vi "Apply UI Theme.vi"(4 "close ref?":bool=TRUE, 6 "save?":bool=TRUE, 7 "VI Refnum":refnum<vi>, 8 "error in":errorcluster, 10 "Theme Mode":u16(ring)=3 items=["Light Theme", "Light Medium Contrast", "Light High Contrast", "Dark Theme", "Dark Medium Contrast", "Dark High Constrast"], 11 "Material Theme in":refnum<class "Material Theme.lvclass">) -> (0 "error out":errorcluster, 3 "Material Theme out":refnum<class "Material Theme.lvclass">)   [LabVIEW 2021, in "TSC Material Theme.lvlib" / "Material Theme.lvclass"]
doc: "Apply a loaded theme to a VI - will update the panel and the controls/indicators\n\n<b>Code Developed By:</b>\nDaniel Coons\nTechnology Service Corporation\nwww.tsc.com/atcs"
uses:
  Material Theme.lvclass
  <vilib>/Utility/traverseref.llb/TRef TravTarget.ctl
  Material Theme.lvclass/Material Theme.ctl
  Material-Scheme/Material-Scheme.lvclass
  <vilib>/Utility/traverseref.llb/VI Scripting - Traverse.lvlib
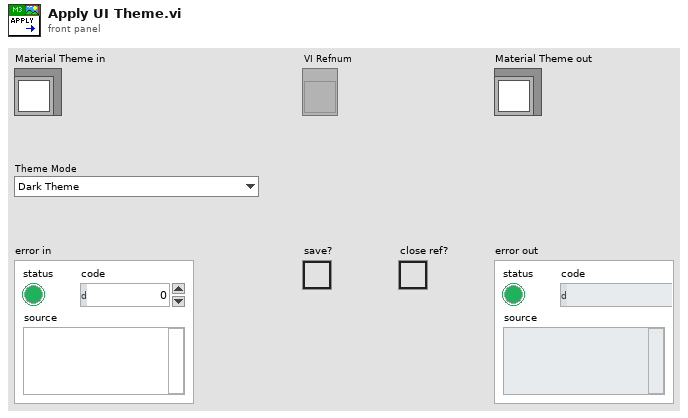
[diagram p1: front panel]
types:
  T1 = typedef "TRef TravTarget.ctl" = enum16{"FP", "BD", "Other"}
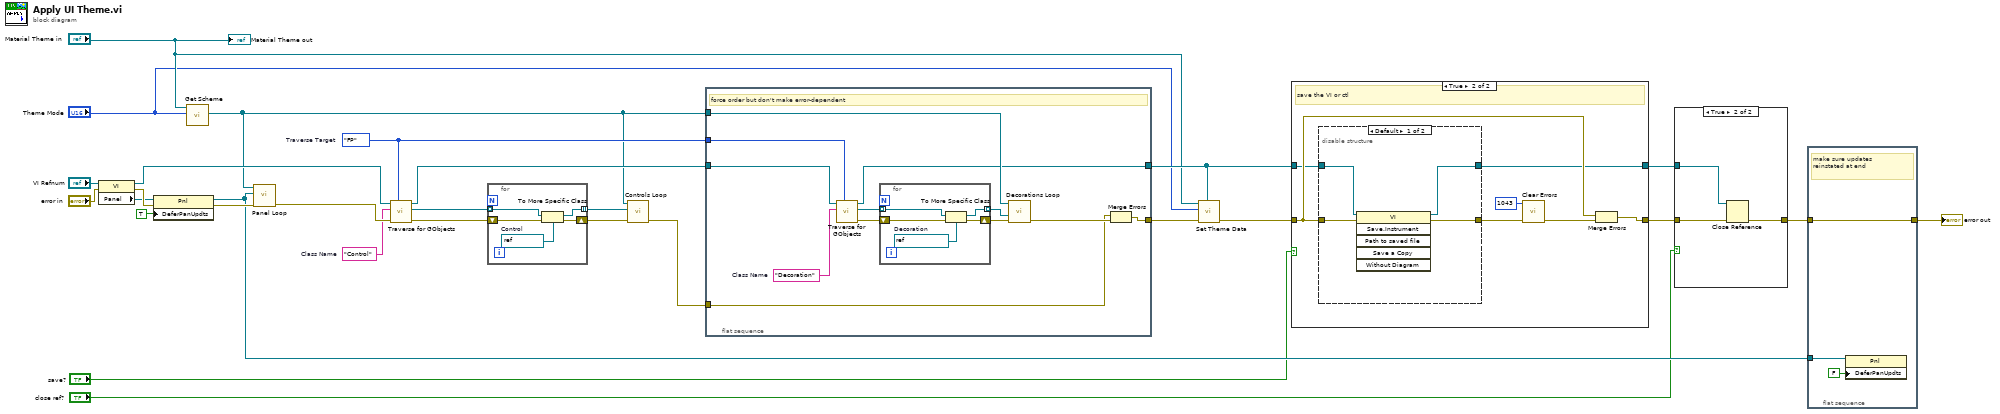
[diagram p0: block diagram]
diagram:
  w5 = TRef_TravTarget."FP"  # Traverse Target
  w9 = "Control"  # Class Name
  n1 = property class="VI"(reference="VI Refnum", error in="error in") -> (reference out=w10:refnum<vi>, error out=w29:errorcluster, "Panel"=w15:refnum<vi>)
  n2 = property class="Pnl"(reference=w15, error in=w29, "DeferPanUpdts"=TRUE ("Defer Panel Updates")) -> (reference out=w14:refnum<vi>, error out=w25:errorcluster)
  n3 = call "Get Scheme.vi"("Theme"="Theme Mode", "Material Theme in"="Material Theme in") -> ("Material-Scheme"=w4:refnum<class "Material-Scheme.lvclass">)  [unwired: 7 in, 2 out]
  n4 = call "Panel Loop.vi"("error in"=w25, "panel"=w14, "Material-Scheme in"=w4) -> ("error out"=w28:errorcluster)  [unwired: 8 in]
  n5 = call <vilib>:"Traverse for GObjects.vi"("Traverse Target"=w5, "error in (no error)"=w28, "Class Name"=w9, "VI Refnum"=w10) -> ("error out"=w22:errorcluster, "References"=w8:refnum<vi>[], "dup VI Refnum"=w6:refnum<vi>)  [unwired: 4 in, 1 out]
  n6 = for {
    tunnel: w8 -> [w31] mode=indexing
    shift-right: [w33] -> w21
    shift-left: w22 -> [w34]
    tunnel: [w30] -> w7 mode=indexing
    w32 = refnum<vi> refnum  # Control
    n7 = To More Specific Class(target class=w32, reference=w31, error in=w34) -> (specific class reference=w30:refnum<vi>, error out=w33:errorcluster)
  }
  n8 = call "Controls Loop.vi"("error in"=w21, "Controls[]"=w7, "Material-Scheme in"=w4) -> ("error out"=w20:errorcluster)  [unwired: 8 in]
  n9 = flat-sequence {
    tunnel: [w45] -> w19
    tunnel: w4 -> [w41]
    tunnel: w6 -> [w40]
    tunnel: w5 -> [w38]
    tunnel: [w37] -> w3
    tunnel: w20 -> [w42]
    frame #0 {
      w39 = "Decoration"  # Class Name
      # "force order but don't make error-dependent"
      n10 = call <vilib>:"Traverse for GObjects.vi"("Traverse Target"=w38, "Class Name"=w39, "VI Refnum"=w40) -> ("error out"=w44:errorcluster, "References"=w36:refnum<vi>[], "dup VI Refnum"=w37:refnum<vi>)  [unwired: 5 in, 1 out]
      n11 = for {
        tunnel: w36 -> [w48] mode=indexing
        shift-right: [w50] -> w43
        shift-left: w44 -> [w51]
        tunnel: [w47] -> w35 mode=indexing
        w49 = refnum<vi> refnum  # Decoration
        n12 = To More Specific Class(target class=w49, reference=w48, error in=w51) -> (specific class reference=w47:refnum<vi>, error out=w50:errorcluster)
      }
      n13 = call "Decorations Loop.vi"("error in (no error)"=w43, "Decos[]"=w35, "Material-Scheme in"=w41) -> ("error out"=w46:errorcluster)  [unwired: 8 in]
      n14 = Merge Errors(w42, w46) -> (w45:errorcluster)
    }
  }
  n15 = call "Set Theme Data.vi"("VI Refnum"=w3, "error in"=w19, "Theme"="Theme Mode", "Material Theme.lvclass"="Material Theme in") -> ("error out"=w18:errorcluster)  [unwired: 7 in]
  n16 = case shown="True" "save?" {
    tunnel: [w53 w59] -> w27
    tunnel: w3 -> [w52 w56]
    tunnel: [w52 w55] -> w16
    tunnel: w18 -> [w53 w58]
    frame False {
    }
    frame True {
      # "save the VI or ctl"
      n17 = disable-structure shown="Default" {
        disable-tunnel: [w64 w66] -> w60
        disable-tunnel: w56 -> [w62 w65]
        disable-tunnel: [w61 w65] -> w55
        disable-tunnel: w58 -> [w63 w66]
        frame condition #0 (active) {
          n18 = invoke class="VI" method="Save.Instrument"(reference=w62, error in=w63) -> (reference out=w61:refnum<vi>, error out=w64:errorcluster)  [unwired: 4 in, 4 out]
        }
        frame condition #1 {
        }
      }
      n19 = call <vilib>:"Clear Errors.vi"("error in (no error)"=w60, "specific error code to clear (0: all)"=1043) -> ("error out"=w57:errorcluster)  [unwired: 4 in, 1 out]
      n20 = Merge Errors(w58, w57) -> (w59:errorcluster)
    }
  }
  n21 = case shown="True" "close ref?" {
    tunnel: w27 -> [w67 w70]
    tunnel: w16 -> [_ w68]
    tunnel: [w67 w69] -> w26
    frame False {
      # "do not want to close reference for Quickdrop"
    }
    frame True {
      n22 = Close Reference(reference=w68, error in (no error)=w70) -> (error out=w69:errorcluster)
    }
  }
  n23 = flat-sequence {
    tunnel: w26 -> [w73]
    tunnel: [w73] -> w23
    tunnel: w14 -> [w72]
    frame #0 {
      # "make sure updates reinstated at end"
      n24 = property class="Pnl"(reference=w72, "DeferPanUpdts"=FALSE ("Defer Panel Updates")) -> ()  [unwired: 1 in, 2 out]
    }
  }
  "error out" <- w23
  "Material Theme out" <- "Material Theme in"
